vi "导通测试.vi"(8 "error in (no error)":errorcluster, 10 "导通阈值":dbl, 11 "仪器实例 in":T1) -> (0 "error out":errorcluster, 1 "导通判断":bool[](array[boolean]), 2 "粘连判断":bool[](array[boolean]), 3 "仪器实例 out":T1, 4 "预充电阻":dbl, 5 "导通值":dbl[](array[numeric]))   [LabVIEW 2020]
uses:
  F:/F020/S7_1200 control/HslCommunication.dll
  S7_1200 control/HslCommunication.dll
  <instrlib>/Keithley 27XX/Public/Data/Read Multiple Direct.vi
  <instrlib>/Keithley 27XX/Keithley 27XX.lvlib
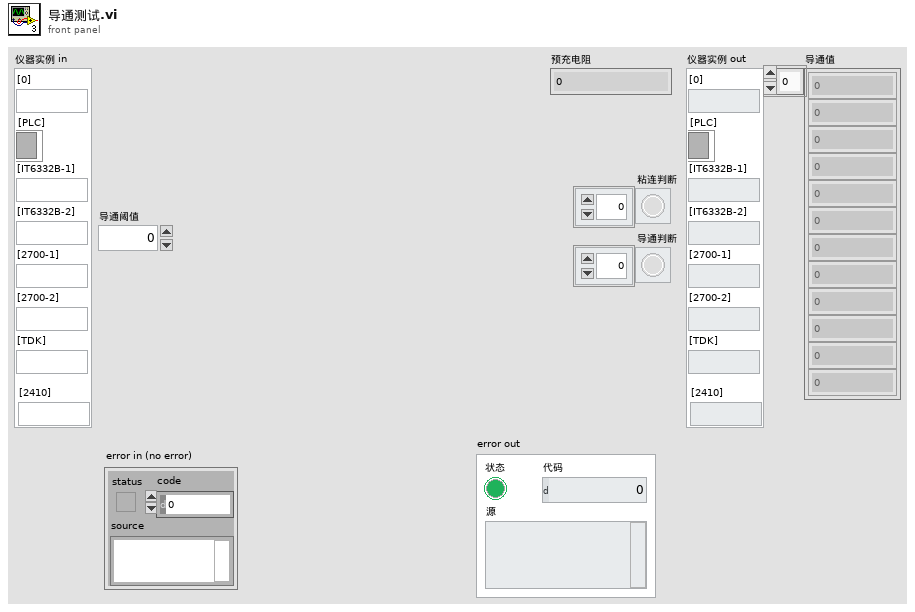
[diagram p1: front panel]
types:
  T1 = typedef "仪器实例.ctl" = cluster{"[0]":string, "[PLC]":refnum<k24>, "[IT6332B-1]":string, "[IT6332B-2]":string, "[2700-1]":string, "[2700-2]":string, "[TDK]":string, "[2410]":string}
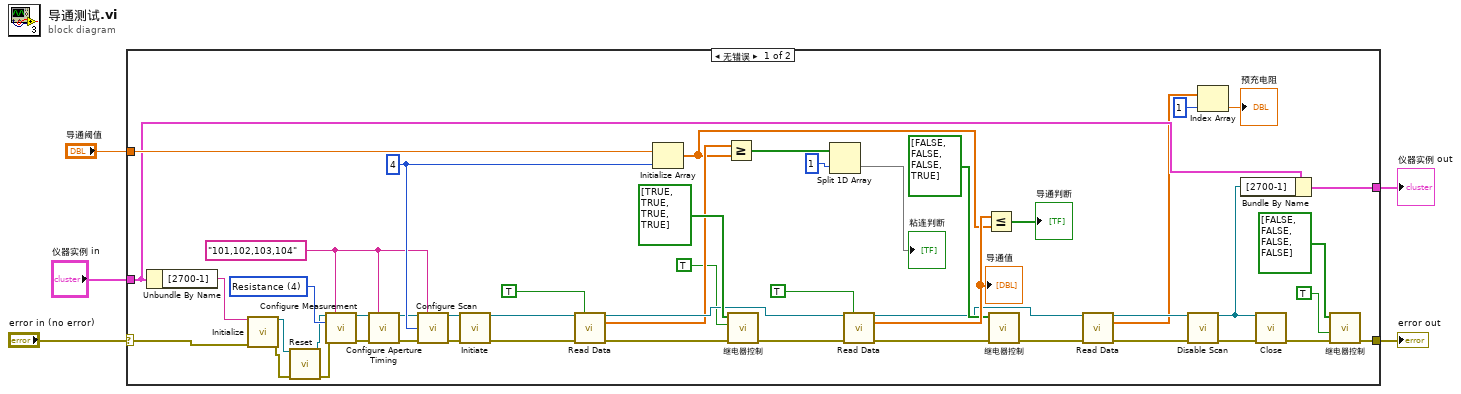
[diagram p0: block diagram]
diagram:
  n1 = case shown="无错误" "error in (no error)" {
    selector: "error in (no error)" -> [w40 w56]
    tunnel: "仪器实例 in" -> [w30 w55]
    tunnel: [w33 w56] -> w4
    tunnel: [w39 w55] -> w1
    tunnel: "导通阈值" -> [w35 _]
    frame No Error {
      w36 = 4 ("Sample Count (100)")
      w12 = "101,102,103,104" ("Scan List (Empty)")
      w54 = u16 4 items=["DC Voltage", "AC Voltage", "DC Current", "AC Current", "Resistance", "Four-Wire Resistance", "Temperature", "Frequency", "Period", "Continuity"] ("Function (0: DC Voltage)")
      n2 = Unbundle By Name(w30) -> ("[2700-1]"=w51:string)
      n3 = call <instrlib>:"Initialize.vi"("VISA resource name"=w51, "error in (no error)"=w40) -> ("VISA resource name out"=w9:refnum<visa-resource-name>, "error out"=w7:errorcluster)  [unwired: 12 in]
      n4 = call <instrlib>:"Reset.vi"("VISA resource name"=w9, "error in (no error)"=w7) -> ("VISA resource name out"=w8:refnum<visa-resource-name>, "error out"=w6:errorcluster)  [unwired: 12 in]
      n5 = call <instrlib>:"Configure Measurement.vi"("VISA resource name"=w8, "Scan List (Empty)"=w12, "Function (0: DC Voltage)"=w54, "error in (no error)"=w6) -> ("VISA resource name out"=w14:refnum<visa-resource-name>, "error out"=w11:errorcluster)  [unwired: 10 in]
      n6 = call <instrlib>:"Configure Aperture Timing.vi"("VISA resource name"=w14, "Scan List (Empty)"=w12, "error in (no error)"=w11) -> ("VISA resource name out"=w13:refnum<visa-resource-name>, "error out"=w10:errorcluster)  [unwired: 11 in]
      n7 = call <instrlib>:"Configure Scan.vi"("VISA resource name"=w13, "Channel List (101:110)"=w12, "Sample Count (100)"=w36, "error in (no error)"=w10) -> ("VISA resource name out"=w16:refnum<visa-resource-name>, "error out"=w15:errorcluster)  [unwired: 10 in]
      n8 = call <instrlib>:"Initiate.vi"("VISA resource name"=w16, "error in (no error)"=w15) -> ("VISA resource name out"=w53:refnum<visa-resource-name>, "error out"=w52:errorcluster)  [unwired: 12 in]
      n9 = call-poly <instrlib>:"Read Data.vi"("VISA resource name"=w53, "All Data Elements (False)"=TRUE, "error in (no error)"=w52) -> ("VISA resource name out"=w47:refnum<visa-resource-name>, "Measurement Data"=w46:dbl[], "error out"=w49:errorcluster)  [unwired: 7 in, 3 out]
      n10 = Initialize Array(w35, w36) -> (w34:dbl[])
      n11 = Greater Or Equal?(x=w46, y=w34) -> (x >= y?=w43:bool[])
      n12 = call "继电器控制.vi"("error in"=w49, "初始化"=TRUE, "继电器控制"=bool[] [TRUE, TRUE, TRUE, TRUE]) -> ("error out"=w48:errorcluster)  [unwired: 8 in]
      n13 = Split 1D Array(array=w43, index=1 ("索引")) -> (second subarray=→"粘连判断":bool[])  [unwired: 1 out]
      n14 = call-poly <instrlib>:"Read Data.vi"("VISA resource name"=w47, "All Data Elements (False)"=TRUE, "error in (no error)"=w48) -> ("VISA resource name out"=w22:refnum<visa-resource-name>, "Measurement Data"=w45:dbl[], "error out"=w25:errorcluster)  [unwired: 7 in, 3 out]
      "导通值" <- w45
      n15 = Less Or Equal?(x=w45, y=w34) -> (x <= y?=→"导通判断":bool[])
      n16 = call "继电器控制.vi"("error in"=w25, "继电器控制"=bool[] [FALSE, FALSE, FALSE, TRUE]) -> ("error out"=w23:errorcluster)  [unwired: 9 in]
      n17 = call-poly <instrlib>:"Read Data.vi"("VISA resource name"=w22, "error in (no error)"=w23) -> ("VISA resource name out"=w21:refnum<visa-resource-name>, "Measurement Data"=w19:dbl[], "error out"=w20:errorcluster)  [unwired: 8 in, 3 out]
      n18 = call <instrlib>:"Disable Scan.vi"("VISA resource name"=w21, "error in (no error)"=w20) -> ("VISA resource name out"=w29:refnum<visa-resource-name>, "error out"=w31:errorcluster)  [unwired: 12 in]
      n19 = Index Array(array=w19, index=1 ("索引")) -> (element=→"预充电阻":dbl)
      n20 = Bundle By Name(cluster=w30, "[2700-1]"=w29) -> (w39:T1)
      n21 = call <instrlib>:"Close.vi"("VISA resource name"=w29, "error in (no error)"=w31) -> ("error out"=w28:errorcluster)  [unwired: 13 in]
      n22 = call "继电器控制.vi"("error in"=w28, "释放"=TRUE, "继电器控制"=bool[] [FALSE, FALSE, FALSE, FALSE]) -> ("error out"=w33:errorcluster)  [unwired: 8 in]
    }
    frame Error {
    }
  }
  "error out" <- w4
  "仪器实例 out" <- w1
